vi "Read Enabled Controllers.vi"(8 "error in (no error)":errorcluster, 11 "Single Channel in":refnum<class "Single Channel.lvclass">) -> (0 "error out":errorcluster, 2 "Enabled Controllers":string[](array[string]), 3 "Single Channel out":refnum<class "Single Channel.lvclass">)   [LabVIEW 2018, in "Single Channel.lvclass"]
doc: "Single Channel.lvclass:Read Enabled Channels.vi\n\nThis VI returns the list of channel names that are enabled for the Single Channel class..\n\nInstrument Communication Module Version 1.0\nOctober, 2020 Original Code Consulting Davita Bird\n www.originalcode.com"
uses:
  Single Channel.lvclass
  Single Channel.lvclass/Single Channel.ctl
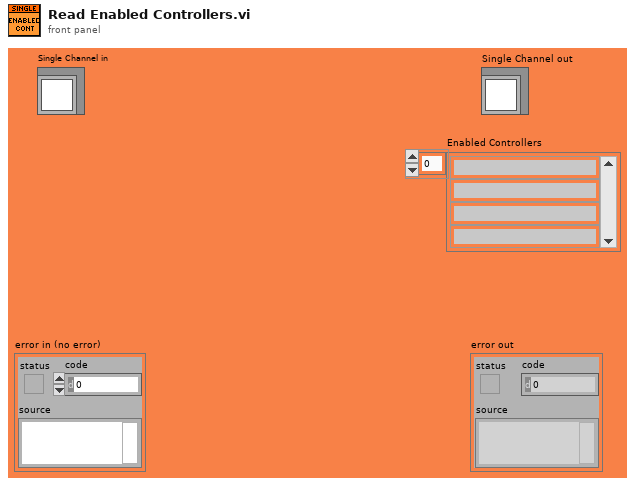
[diagram p1: front panel]
types:
  T1 = cluster{"Parsing String":string, "Channel Name":string, "Enabled":bool, "Initial Value":dbl}[]
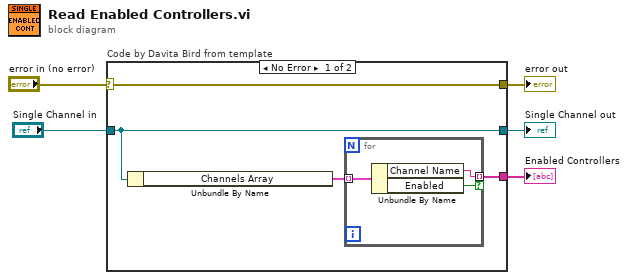
[diagram p0: block diagram]
diagram:
  n1 = case "Code by Davita Bird from template" shown="No Error" "error in (no error)" {
    selector: "error in (no error)" -> [w9 w13]
    tunnel: [w9 w13] -> w4
    tunnel: [w8 w14] -> w1
    tunnel: "Single Channel in" -> [w8 w14]
    tunnel: [w6 _] -> w3
    frame No Error {
      n2 = Unbundle By Name(w8) -> ("Channels Array"=w7:T1)
      n3 = for {
        tunnel: [w11] -> w6 mode=indexing if=w10
        tunnel: w7 -> [w12] mode=indexing
        n4 = Unbundle By Name(w12) -> ("Channel Name"=w11:string, "Enabled"=w10:bool)
      }
    }
    frame Error {
    }
  }
  "error out" <- w4
  "Enabled Controllers" <- w3
  "Single Channel out" <- w1
